vi "Moving Average Filter.vi"(10 "Input 2":dbl, 11 "Input":dbl) -> (2 "Filtered2":dbl, 3 "Filtered":dbl)   [LabVIEW 2013, in "main.lvlib"]
uses:
  main.lvlib
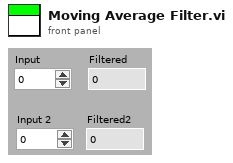
[diagram p1: front panel]
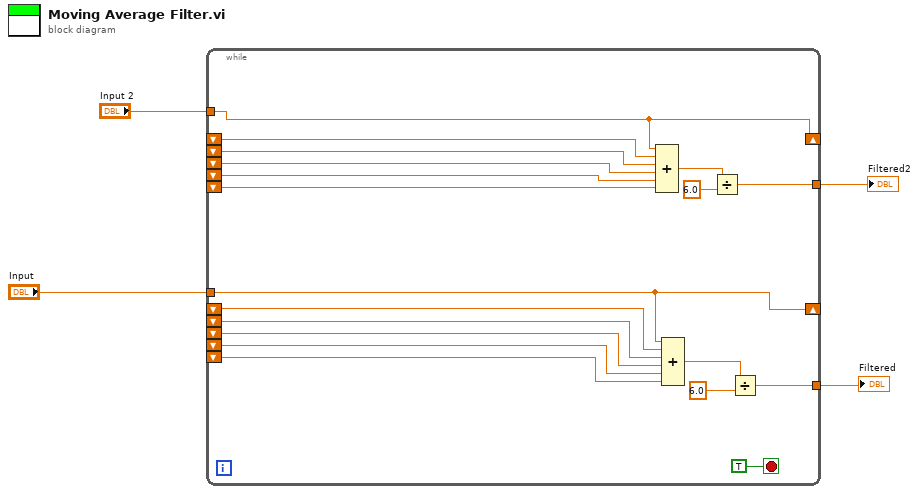
[diagram p0: block diagram]
diagram:
  n1 = while {
    shift-right: [w22] -> _
    shift-left: _ -> [w23]
    tunnel: "Input" -> [w22]
    tunnel: [w20] -> w3
    shift-left: _ -> [w19]
    shift-right: [w18] -> _
    shift-left: _ -> [w17]
    tunnel: "Input 2" -> [w18]
    shift-left: _ -> [w16]
    tunnel: [w15] -> w1
    shift-left: _ -> [w11]
    shift-left: _ -> [w10]
    shift-left: _ -> [w14]
    shift-left: _ -> [w13]
    shift-left: _ -> [w12]
    shift-left: _ -> [w9]
    stop <- TRUE stop-if-true
    n2 = Compound Arithmetic op=ADD(w18, w17, w16, w11, w10, w9) -> (w6:dbl)
    n3 = Compound Arithmetic op=ADD(w22, w23, w19, w14, w13, w12) -> (w8:dbl)
    n4 = Divide(x=w6, y=6.0) -> (x/y=w15:dbl)
    n5 = Divide(x=w8, y=6.0) -> (x/y=w20:dbl)
  }
  "Filtered" <- w3
  "Filtered2" <- w1
